vi "Set Roller Orientation.vi"(8 "error in (no error)":errorcluster, 10 "roller orientation":T1 items=["Left", "Right"], 11 "mecanum wheel in":refnum<class "NI_Robotics_Mecanum Wheel.lvclass">) -> (0 "error out":errorcluster, 3 "mecanum wheel out":refnum<class "NI_Robotics_Mecanum Wheel.lvclass">)   [LabVIEW 2017, in "NI_Robotics_Mecanum Wheel.lvclass"]
uses:
  <vilib>/robotics/Steering/Mecanum Wheel/NI_Robotics_Mecanum Wheel.lvclass
  <vilib>/robotics/Steering/Mecanum Wheel/Roller Orientation.ctl
  <vilib>/robotics/Steering/Mecanum Wheel/NI_Robotics_Mecanum Wheel.lvclass/NI_Robotics_Mecanum Wheel.ctl
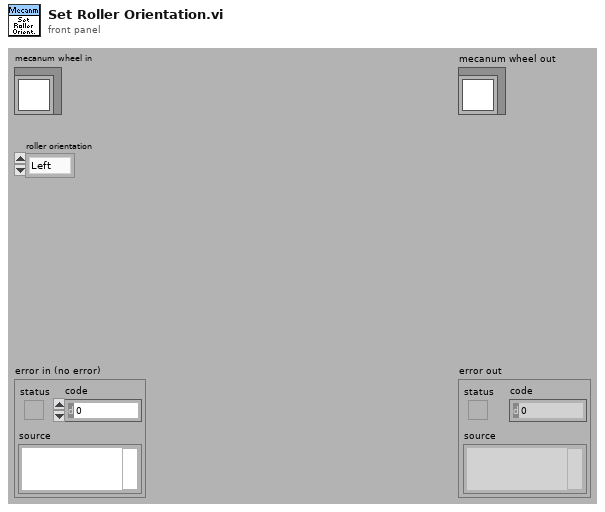
[diagram p1: front panel]
types:
  T1 = typedef "NI_Robotics_Mecanum Wheel.lvclass/Roller Orientation.ctl" = u16
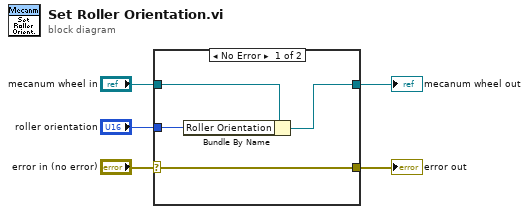
[diagram p0: block diagram]
diagram:
  n1 = case shown="No Error" "error in (no error)" {
    selector: "error in (no error)" -> [w9 w10]
    tunnel: [w9 w10] -> w4
    tunnel: [w7 w11] -> w2
    tunnel: "mecanum wheel in" -> [w8 w11]
    tunnel: "roller orientation" -> [w6 _]
    frame No Error {
      n2 = Bundle By Name(cluster=w8, "Roller Orientation"=w6) -> (w7:refnum<class "NI_Robotics_Mecanum Wheel.lvclass">)
    }
    frame Error {
    }
  }
  "error out" <- w4
  "mecanum wheel out" <- w2
